vi "Instrument Type ID.vi"() -> (1 "instrument type id":string="niDMM")   [LabVIEW 2020, in "MeasurementLink niDMM.lvlib"]
uses:
  MeasurementLink niDMM.lvlib
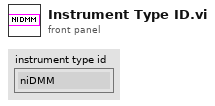
[diagram p1: front panel]
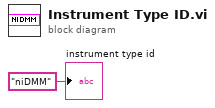
[diagram p0: block diagram]
diagram:
  "instrument type id" <- "niDMM" ("instrument type id")
